vi "Cross product 3D_3Dpf.vi"(1 "B":sgl[](array[numeric]), 2 "A":sgl[](array[numeric])) -> (0 "A x B":sgl[](array[numeric]))   [LabVIEW 2017]
panel:
  # "PN 13/01/2015"
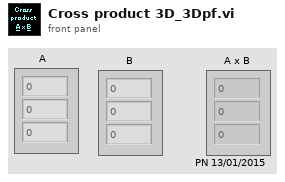
[diagram p1: front panel]
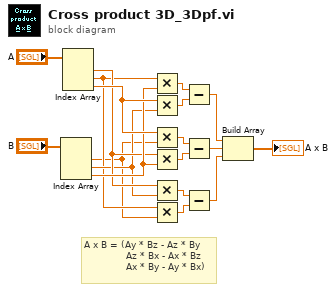
[diagram p0: block diagram]
diagram:
  # "A x B = (Ay * Bz - Az * By\n              Az * Bx - Ax * Bz\n              Ax * By - Ay * Bx)"
  n1 = Index Array(array="B") -> (element #1=w3:sgl, element #2=w6:sgl, element #3=w11:sgl)  [unwired: 3 in]
  n2 = Index Array(array="A") -> (element #1=w7:sgl, element #2=w4:sgl, element #3=w12:sgl)  [unwired: 3 in]
  n3 = Multiply(x=w4, y=w11) -> (x*y=w15:sgl)
  n4 = Multiply(x=w12, y=w6) -> (x*y=w14:sgl)
  n5 = Multiply(x=w12, y=w3) -> (x*y=w10:sgl)
  n6 = Multiply(x=w7, y=w11) -> (x*y=w9:sgl)
  n7 = Multiply(x=w7, y=w6) -> (x*y=w5:sgl)
  n8 = Multiply(x=w4, y=w3) -> (x*y=w2:sgl)
  n9 = Subtract(x=w15, y=w14) -> (x-y=w13:sgl)
  n10 = Subtract(x=w10, y=w9) -> (x-y=w8:sgl)
  n11 = Subtract(x=w5, y=w2) -> (x-y=w1:sgl)
  n12 = Build Array(w13, w8, w1) -> (→"A x B":sgl[])
